vi "Control AlgorithmV2.vi"(5 "Motor to Control":dbl, 8 "Manual Control":bool, 9 "Angles In":dbl[](array[numeric]), 10 "JoystickIn":i32[](array[numeric])) -> (2 "Target Angles":dbl[](array[numeric]), 3 "MotorsOut":u16[](array[numeric]))   [LabVIEW 2013, in "ProcessorHelperFunctions.lvlib"]
uses:
  ProcessorHelperFunctions.lvlib
panel:
  in  "D gain":dbl
  in  "I Gain":dbl
  in  "Pgain":dbl=1.5
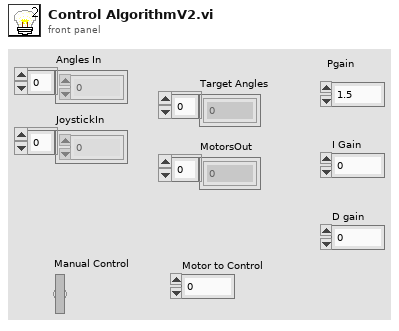
[diagram p1: front panel]
types:
  T1 = cluster{"JoystickIn[0]":i32, "JoystickIn[1]":i32, "JoystickIn[2]":i32, "JoystickIn[3]":i32, "JoystickIn[4]":i32, "JoystickIn[5]":i32, "JoystickIn[6]":i32, "JoystickIn[7]":i32, "JoystickIn[8]":i32, "JoystickIn[9]":i32}
  T2 = cluster{"Angles In[0]":dbl, "Angles In[1]":dbl, "Angles In[2]":dbl, "Angles In[3]":dbl}
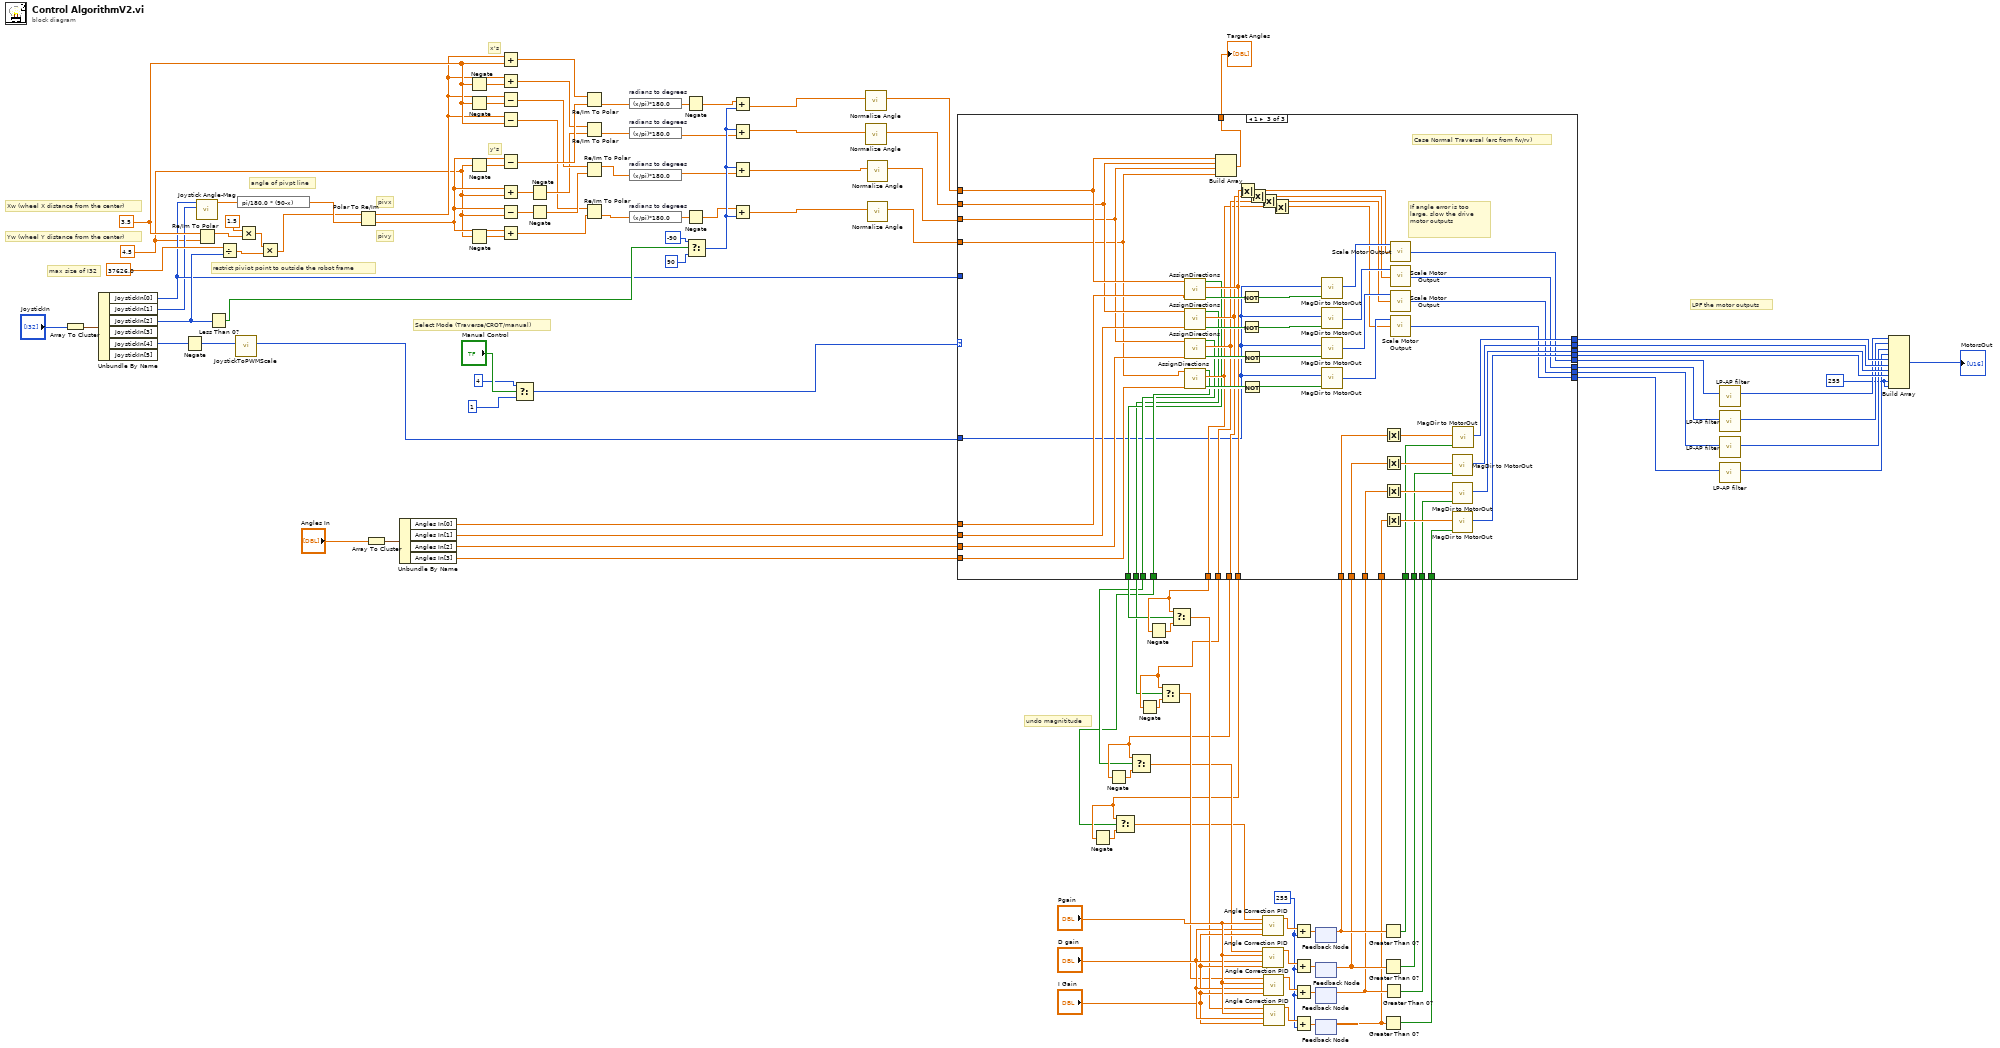
[diagram p0: block diagram]
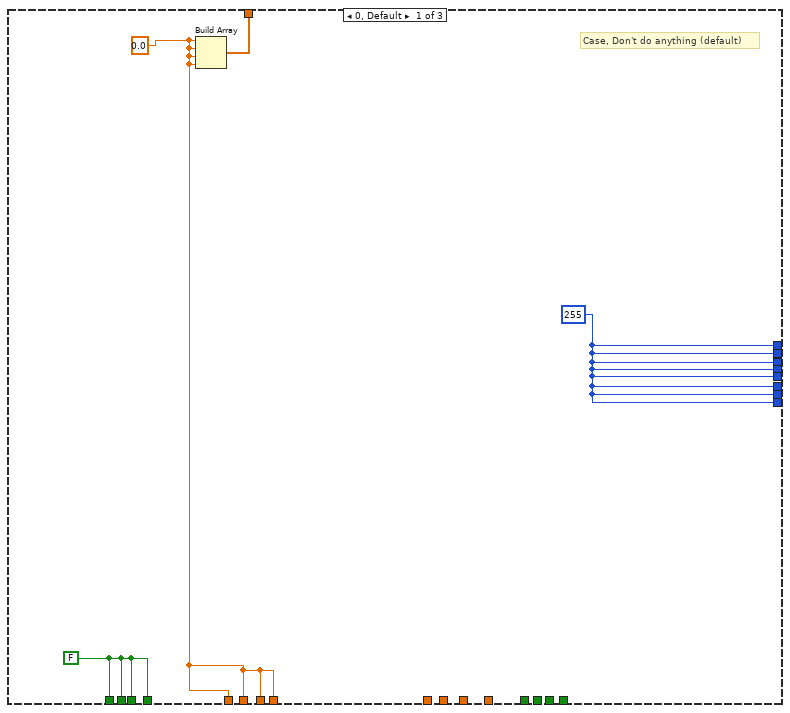
[diagram p2: hidden frame]
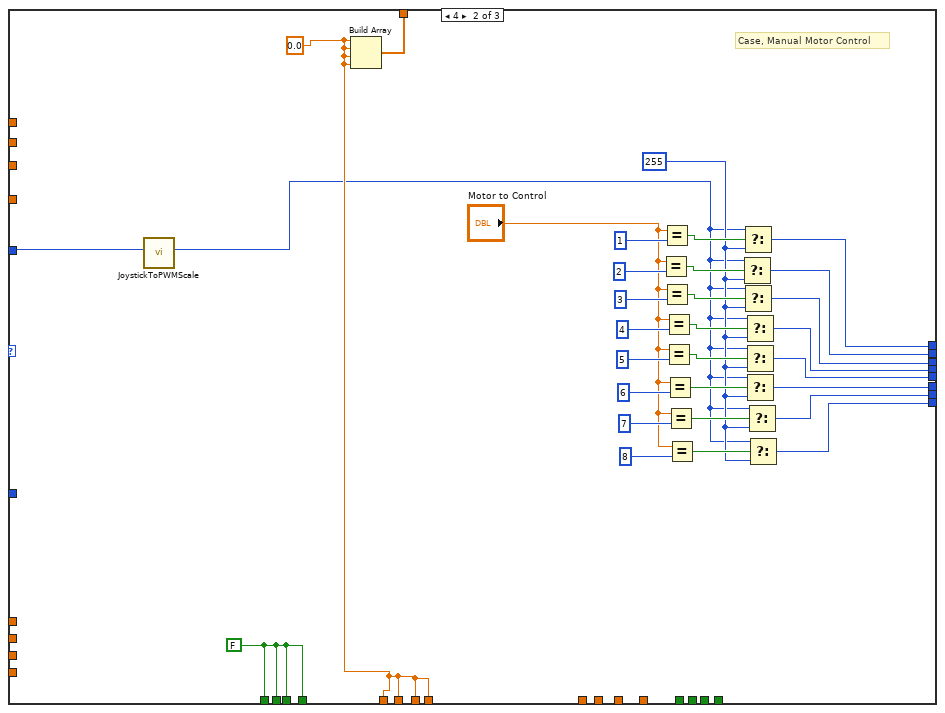
[diagram p3: hidden frame]
diagram:
  w1 = 255
  w32 = 4.5
  w71 = 3.5
  w19 = 255
  # "max size of I32"
  # "y's"
  # "x's"
  # "restrict piviot point to outside the robot frame"
  # "Yw (wheel Y distance from the center)"
  # "Xw (wheel X distance from the center)"
  # "pivy"
  # "pivx"
  # "angle of pivpt line"
  # "undo magnititude"
  # "LPF the motor outputs"
  # "Select Mode (Traverse/CROT/manual)"
  n1 = Array To Cluster(array="JoystickIn") -> (cluster=w116:T1)
  n2 = Unbundle By Name(w116) -> ("JoystickIn[0]"=w54:i32, "JoystickIn[1]"=w53:i32, "JoystickIn[2]"=w66:i32, "JoystickIn[4]"=w68:i32)  [unwired: 2 out]
  n3 = Negate(x=w68) -> (-x=w61:i32)
  n4 = call "Joystick Angle-Mag.vi"("Yaxis"=w53, "Xaxis"=w54) -> ("Angle"=w76:dbl)  [unwired: 8 in, 1 out]
  n5 = Re/Im To Polar(2:w32, 3:w71) -> (1:w74:dbl)  [unwired: 1 out]
  n6 = Less Than 0?(x=w66) -> (x < 0?=w62:bool)
  n7 = Divide(x=37626.0, y=w66) -> (x/y=w70:dbl)
  n8 = call "JoystickToPWMScale.vi"("Numeric"=w61) -> ("Numeric 2"=w67:u16)  [unwired: 10 in]
  n9 = expression code="pi/180.0 * (90-x)"(w76) -> (w77:dbl)
  n10 = Multiply(x=1.5, y=w74) -> (x*y=w60:dbl)
  n11 = Multiply(x=w60, y=w70) -> (x*y=w75:dbl)
  n12 = Polar To Re/Im(2:w77, 3:w75) -> (0:w51:dbl, 1:w52:dbl)
  n13 = Array To Cluster(array="Angles In") -> (cluster=w115:T2)
  n14 = Unbundle By Name(w115) -> ("Angles In[0]"=w113:dbl, "Angles In[1]"=w112:dbl, "Angles In[2]"=w111:dbl, "Angles In[3]"=w110:dbl)
  n15 = Negate(x=w71) -> (-x=w31:dbl)
  n16 = Negate(x=w71) -> (-x=w30:dbl)
  n17 = Negate(x=w32) -> (-x=w29:dbl)
  n18 = Negate(x=w32) -> (-x=w28:dbl)
  n19 = Add(x=w52, y=w71) -> (x+y=w26:dbl)
  n20 = Add(x=w52, y=w31) -> (x+y=w38:dbl)
  n21 = Subtract(x=w52, y=w30) -> (x-y=w37:dbl)
  n22 = Subtract(x=w52, y=w71) -> (x-y=w27:dbl)
  n23 = Subtract(x=w51, y=w29) -> (x-y=w73:dbl)
  n24 = Add(x=w51, y=w32) -> (x+y=w36:dbl)
  n25 = Subtract(x=w51, y=w32) -> (x-y=w35:dbl)
  n26 = Add(x=w51, y=w28) -> (x+y=w72:dbl)
  n27 = Select(t=4, s="Manual Control", f=1) -> (s? t:f=w108:i32)
  n28 = Negate(x=w36) -> (-x=w34:dbl)
  n29 = Negate(x=w35) -> (-x=w33:dbl)
  n30 = Re/Im To Polar(2:w73, 3:w26) -> (0:w58:dbl)  [unwired: 1 out]
  n31 = Re/Im To Polar(2:w34, 3:w38) -> (0:w57:dbl)  [unwired: 1 out]
  n32 = Re/Im To Polar(2:w33, 3:w37) -> (0:w56:dbl)  [unwired: 1 out]
  n33 = Re/Im To Polar(2:w72, 3:w27) -> (0:w55:dbl)  [unwired: 1 out]
  n34 = expression code="(x/pi)*180.0" "radians to degrees"(w58) -> (w42:dbl)
  n35 = expression code="(x/pi)*180.0" "radians to degrees"(w57) -> (w41:dbl)
  n36 = expression code="(x/pi)*180.0" "radians to degrees"(w56) -> (w40:dbl)
  n37 = expression code="(x/pi)*180.0" "radians to degrees"(w55) -> (w39:dbl)
  n38 = Negate(x=w42) -> (-x=w25:dbl)
  n39 = Negate(x=w39) -> (-x=w24:dbl)
  n40 = Select(t=-90, s=w62, f=90) -> (s? t:f=w65:i32)
  n41 = Add(x=w25, y=w65) -> (x+y=w50:dbl)
  n42 = Add(x=w65, y=w41) -> (x+y=w47:dbl)
  n43 = Add(x=w65, y=w40) -> (x+y=w48:dbl)
  n44 = Add(x=w24, y=w65) -> (x+y=w49:dbl)
  n45 = call "Normalize Angle.vi"("Input"=w50) -> ("Output"=w46:dbl)  [unwired: 10 in]
  n46 = call "Normalize Angle.vi"("Input"=w47) -> ("Output"=w45:dbl)  [unwired: 10 in]
  n47 = call "Normalize Angle.vi"("Input"=w48) -> ("Output"=w44:dbl)  [unwired: 10 in]
  n48 = call "Normalize Angle.vi"("Input"=w49) -> ("Output"=w43:dbl)  [unwired: 10 in]
  n49 = feedback #1() -> (w18:dbl)  [unwired: 1 in]
  n50 = feedback #2() -> (w17:dbl)  [unwired: 1 in]
  n51 = feedback #3() -> (w16:dbl)  [unwired: 1 in]
  n52 = feedback #4() -> (w15:dbl)  [unwired: 1 in]
  n53 = Greater Than 0?(x=w18) -> (x > 0?=w14:bool)
  n54 = Greater Than 0?(x=w17) -> (x > 0?=w13:bool)
  n55 = Greater Than 0?(x=w15) -> (x > 0?=w11:bool)
  n56 = Greater Than 0?(x=w16) -> (x > 0?=w12:bool)
  n57 = case shown="1" w108 {
    tunnel: [w121 w149 w202] -> w9
    tunnel: [w121 w134 w201] -> w8
    tunnel: [w121 w133 w200] -> w7
    tunnel: [w121 w132 w199] -> w6
    tunnel: [w121 w131 w170] -> w105
    tunnel: [w121 w130 w169] -> w104
    tunnel: [w121 w129 w168] -> w103
    tunnel: [w121 w128 w167] -> w102
    tunnel: w113 -> [_ _ w190]
    tunnel: w112 -> [_ _ w189]
    tunnel: w111 -> [_ _ w188]
    tunnel: w110 -> [_ _ w187]
    tunnel: w54 -> [_ w123 _]
    tunnel: [w120 w152 w186] -> w109
    tunnel: [w119 w125 w185] -> w79
    tunnel: [w119 w125 w184] -> w83
    tunnel: [w119 w125 w183] -> w86
    tunnel: [w119 w125 w182] -> w89
    tunnel: w18 -> [_ _ w181]
    tunnel: w17 -> [_ _ w180]
    tunnel: w16 -> [_ _ w179]
    tunnel: w15 -> [_ _ w178]
    tunnel: [w118 w124 w177] -> w20
    tunnel: [w118 w124 w176] -> w21
    tunnel: [w118 w124 w174] -> w22
    tunnel: [w118 w124 w175] -> w23
    tunnel: w67 -> [_ _ w165]
    tunnel: w46 -> [_ _ w164]
    tunnel: w45 -> [_ _ w163]
    tunnel: w44 -> [_ _ w162]
    tunnel: w43 -> [_ _ w161]
    tunnel: w14 -> [_ _ w156]
    tunnel: w13 -> [_ _ w155]
    tunnel: w12 -> [_ _ w154]
    tunnel: w11 -> [_ _ w153]
    frame 0, Default {
      w118 = FALSE
      w119 = 0.0
      w121 = 255
      # "Case, Don't do anything (default)"
      n58 = Build Array(w119, w119, w119, w119) -> (w120:dbl[])
    }
    frame 4 {
      w124 = FALSE
      w127 = 255
      w125 = 0.0
      # "Case, Manual Motor Control"
      n59 = call "JoystickToPWMScale.vi"("Numeric"=w123) -> ("Numeric 2"=w122:u16)  [unwired: 10 in]
      n60 = Build Array(w125, w125, w125, w125) -> (w152:dbl[])
      n61 = Equal?(x="Motor to Control", y=2) -> (x = y?=w147:bool)
      n62 = Equal?(x="Motor to Control", y=1) -> (x = y?=w150:bool)
      n63 = Equal?(x="Motor to Control", y=3) -> (x = y?=w145:bool)
      n64 = Equal?(x="Motor to Control", y=4) -> (x = y?=w143:bool)
      n65 = Equal?(x="Motor to Control", y=5) -> (x = y?=w141:bool)
      n66 = Equal?(x="Motor to Control", y=6) -> (x = y?=w139:bool)
      n67 = Equal?(x="Motor to Control", y=7) -> (x = y?=w137:bool)
      n68 = Equal?(x="Motor to Control", y=8) -> (x = y?=w135:bool)
      n69 = Select(t=w122, s=w147, f=w127) -> (s? t:f=w134:i32)
      n70 = Select(t=w122, s=w150, f=w127) -> (s? t:f=w149:i32)
      n71 = Select(t=w122, s=w145, f=w127) -> (s? t:f=w133:i32)
      n72 = Select(t=w122, s=w143, f=w127) -> (s? t:f=w132:i32)
      n73 = Select(t=w122, s=w141, f=w127) -> (s? t:f=w131:i32)
      n74 = Select(t=w122, s=w139, f=w127) -> (s? t:f=w130:i32)
      n75 = Select(t=w122, s=w137, f=w127) -> (s? t:f=w129:i32)
      n76 = Select(t=w122, s=w135, f=w127) -> (s? t:f=w128:i32)
    }
    frame 1 {
      # "Case Normal Traversal (arc from fw/rv)"
      # "If angle error is too large, slow the drive motor outputs"
      n77 = call "AssignDirections.vi"("Actual Angle"=w190, "Target Angle"=w164) -> ("Reverse Wheel Direction"=w206:bool, "Lowest Angle Error"=w185:dbl, "Turn Clockwise"=w175:bool)  [unwired: 7 in]
      n78 = call "AssignDirections.vi"("Actual Angle"=w189, "Target Angle"=w163) -> ("Reverse Wheel Direction"=w205:bool, "Lowest Angle Error"=w184:dbl, "Turn Clockwise"=w174:bool)  [unwired: 7 in]
      n79 = call "AssignDirections.vi"("Actual Angle"=w188, "Target Angle"=w162) -> ("Reverse Wheel Direction"=w204:bool, "Lowest Angle Error"=w183:dbl, "Turn Clockwise"=w176:bool)  [unwired: 7 in]
      n80 = call "AssignDirections.vi"("Actual Angle"=w187, "Target Angle"=w161) -> ("Reverse Wheel Direction"=w203:bool, "Lowest Angle Error"=w182:dbl, "Turn Clockwise"=w177:bool)  [unwired: 7 in]
      n81 = Build Array(w164, w163, w162, w161) -> (w186:dbl[])
      n82 = Absolute Value(x=w185) -> (abs(x)=w173:dbl)
      n83 = Not(x=w206) -> (.not. x?=w191:bool)
      n84 = Not(x=w205) -> (.not. x?=w192:bool)
      n85 = Not(x=w204) -> (.not. x?=w193:bool)
      n86 = Not(x=w203) -> (.not. x?=w194:bool)
      n87 = Absolute Value(x=w184) -> (abs(x)=w166:dbl)
      n88 = Absolute Value(x=w183) -> (abs(x)=w172:dbl)
      n89 = Absolute Value(x=w182) -> (abs(x)=w171:dbl)
      n90 = call "MagDir to MotorOut.vi"("Fwd. Dir?"=w191, "Input"=w165) -> ("Output"=w198:i16)  [unwired: 9 in]
      n91 = call "MagDir to MotorOut.vi"("Fwd. Dir?"=w192, "Input"=w165) -> ("Output"=w197:i16)  [unwired: 9 in]
      n92 = call "MagDir to MotorOut.vi"("Fwd. Dir?"=w193, "Input"=w165) -> ("Output"=w196:i16)  [unwired: 9 in]
      n93 = call "MagDir to MotorOut.vi"("Fwd. Dir?"=w194, "Input"=w165) -> ("Output"=w195:i16)  [unwired: 9 in]
      n94 = Absolute Value(x=w181) -> (abs(x)=w160:dbl)
      n95 = Absolute Value(x=w180) -> (abs(x)=w159:dbl)
      n96 = Absolute Value(x=w179) -> (abs(x)=w158:dbl)
      n97 = Absolute Value(x=w178) -> (abs(x)=w157:dbl)
      n98 = call "Scale Motor Output.vi"("Error Input"=w173, "Motor Input"=w198) -> ("Output"=w170:u32)  [unwired: 1 in]
      n99 = call "Scale Motor Output.vi"("Error Input"=w166, "Motor Input"=w197) -> ("Output"=w169:u32)  [unwired: 1 in]
      n100 = call "Scale Motor Output.vi"("Error Input"=w172, "Motor Input"=w196) -> ("Output"=w168:u32)  [unwired: 1 in]
      n101 = call "Scale Motor Output.vi"("Error Input"=w171, "Motor Input"=w195) -> ("Output"=w167:u32)  [unwired: 1 in]
      n102 = call "MagDir to MotorOut.vi"("Fwd. Dir?"=w155, "Input"=w159) -> ("Output"=w201:i16)  [unwired: 9 in]
      n103 = call "MagDir to MotorOut.vi"("Fwd. Dir?"=w154, "Input"=w158) -> ("Output"=w200:i16)  [unwired: 9 in]
      n104 = call "MagDir to MotorOut.vi"("Fwd. Dir?"=w153, "Input"=w157) -> ("Output"=w199:i16)  [unwired: 9 in]
      n105 = call "MagDir to MotorOut.vi"("Fwd. Dir?"=w156, "Input"=w160) -> ("Output"=w202:i16)  [unwired: 9 in]
    }
  }
  "Target Angles" <- w109
  n106 = Negate(x=w79) -> (-x=w81:dbl)
  n107 = Negate(x=w83) -> (-x=w84:dbl)
  n108 = Select(t=w79, s=w20, f=w81) -> (s? t:f=w80:dbl)
  n109 = Select(t=w83, s=w21, f=w84) -> (s? t:f=w82:dbl)
  n110 = Negate(x=w86) -> (-x=w87:dbl)
  n111 = Negate(x=w89) -> (-x=w90:dbl)
  n112 = Select(t=w86, s=w22, f=w87) -> (s? t:f=w85:dbl)
  n113 = Select(t=w89, s=w23, f=w90) -> (s? t:f=w88:dbl)
  n114 = call "Angle Correction PID.vi"("I gain"="I Gain", "D gain"="D gain", "P gain"="Pgain", "Error In"=w80) -> ("Output"=w97:dbl)  [unwired: 7 in]
  n115 = call "Angle Correction PID.vi"("I gain"="I Gain", "D gain"="D gain", "P gain"="Pgain", "Error In"=w82) -> ("Output"=w96:dbl)  [unwired: 7 in]
  n116 = call "Angle Correction PID.vi"("I gain"="I Gain", "D gain"="D gain", "P gain"="Pgain", "Error In"=w85) -> ("Output"=w95:dbl)  [unwired: 7 in]
  n117 = call "Angle Correction PID.vi"("I gain"="I Gain", "D gain"="D gain", "P gain"="Pgain", "Error In"=w88) -> ("Output"=w94:dbl)  [unwired: 7 in]
  n118 = Add(x=w97, y=w19) -> (x+y=w101:dbl)
  n119 = Add(x=w96, y=w19) -> (x+y=w100:dbl)
  n120 = Add(x=w95, y=w19) -> (x+y=w99:dbl)
  n121 = Add(x=w94, y=w19) -> (x+y=w98:dbl)
  n122 = feedback-in #1(w101) -> ()
  n123 = feedback-in #2(w100) -> ()
  n124 = feedback-in #3(w99) -> ()
  n125 = feedback-in #4(w98) -> ()
  n126 = call "LP-AP filter.vi"("Input"=w105) -> ("Output"=w5:u16)  [unwired: 9 in, 1 out]
  n127 = call "LP-AP filter.vi"("Input"=w104) -> ("Output"=w4:u16)  [unwired: 9 in, 1 out]
  n128 = call "LP-AP filter.vi"("Input"=w103) -> ("Output"=w3:u16)  [unwired: 9 in, 1 out]
  n129 = call "LP-AP filter.vi"("Input"=w102) -> ("Output"=w2:u16)  [unwired: 9 in, 1 out]
  n130 = Build Array(w5, w4, w3, w2, w9, w8, w7, w6, w1, w1) -> (→"MotorsOut":i32[])
